vi "Read Client status.vi"(8 "error in (no error)":errorcluster, 11 "PD-Main in":refnum<class "PD-Main.lvclass">) -> (0 "error out":errorcluster, 2 "Client status":refnum<vi>, 3 "PD-Main out":refnum<class "PD-Main.lvclass">)   [LabVIEW 2013, in "PowderDeposition.lvlib" / "PD-Main.lvclass"]
uses:
  PD-Main.lvclass
  PD-Main.lvclass/PD-Main.ctl
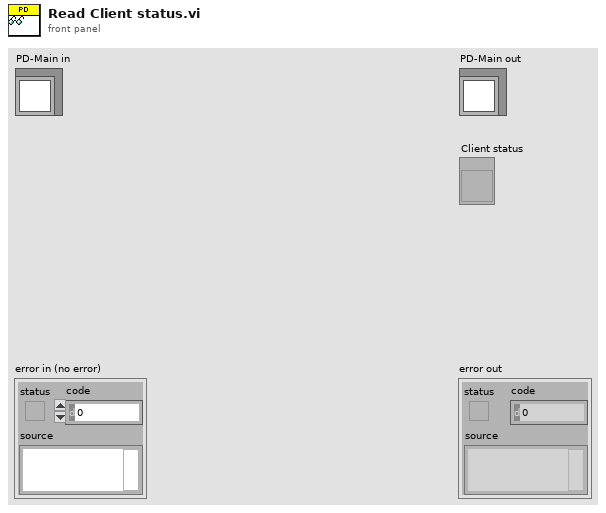
[diagram p1: front panel]
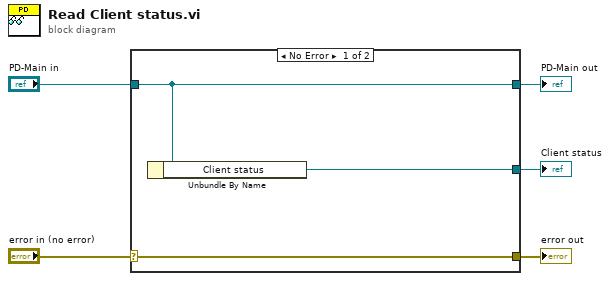
[diagram p0: block diagram]
diagram:
  n1 = case shown="No Error" "error in (no error)" {
    selector: "error in (no error)" -> [w8 w9]
    tunnel: [w8 w9] -> w4
    tunnel: [w7 w10] -> w2
    tunnel: "PD-Main in" -> [w7 w10]
    tunnel: [w6 _] -> w1
    frame No Error {
      n2 = Unbundle By Name(w7) -> ("Client status"=w6:refnum<vi>)
    }
    frame Error {
    }
  }
  "error out" <- w4
  "PD-Main out" <- w2
  "Client status" <- w1
